vi "Window Mini.vi"(8 "error in (no error)":errorcluster, 11 "last level":i32=2) -> (0 "error out":errorcluster)   [LabVIEW 2020]
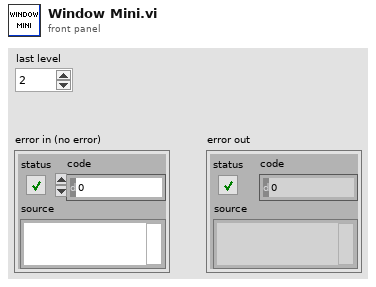
[diagram p1: front panel]
types:
  T1 = enum32{"Invalid", "Standard", "Closed", "Hidden", "Minimized", "Maximized"}
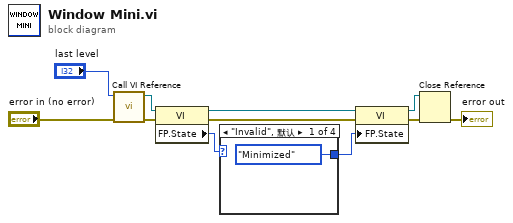
[diagram p0: block diagram]
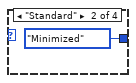
[diagram p2: hidden frame]
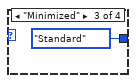
[diagram p3: hidden frame]
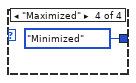
[diagram p4: hidden frame]
diagram:
  n1 = call "Call VI Reference.vi"("error in"="error in (no error)", "last level"="last level") -> ("error out"=w8:errorcluster, "vi reference out"=w11:refnum<vi>)  [unwired: 8 in]
  n2 = property class="VI"(reference=w11, error in=w8) -> (reference out=w9:refnum<vi>, error out=w7:errorcluster, "FP.State"=w10:T1)
  n3 = case shown="\"Invalid\", 默认" w10 {
    tunnel: [T1."Minimized" ("前面板窗口:状态") T1."Minimized" ("前面板窗口:状态") T1."Standard" ("前面板窗口:状态") T1."Minimized" ("前面板窗口:状态")] -> w4
    frame "Invalid", Default {
    }
    frame "Standard" {
    }
    frame "Minimized" {
    }
    frame "Maximized" {
    }
  }
  n4 = property class="VI"(reference=w9, error in=w7, "FP.State"=w4) -> (reference out=w6:refnum<vi>, error out=w5:errorcluster)
  n5 = Close Reference(reference=w6, error in (no error)=w5) -> (error out=→"error out":errorcluster)
